vi "MultRRTPlan.vi"(7 "Parameters.lvclass":refnum<class "Parameters.lvclass">, 8 "Volta ao redor\nda área?":bool, 9 "Line?":bool, 10 "IA State":T7={"our_robots"=[], "enemy_robots"=[], "balls"=[], "geometry"={"line_width"=0, "field_length"=0, "field_width"=0, "boundary_width"=0, "referee_width"=0, "goal_width"=0, "goal_depth"=0, "goal_wall_width"=0, "center_circle_radius"=0, "defense_radius"=0, "defense_stretch"=0, "free_kick_from_defense_dist"=0, "penalty_spot_from_field_line_dist"=0, "penalty_line_from_spot_dist"=0}, "IA Judge"={"stage"="", "command"="", "our_goalie_id"=0.0, "enemy_goalie_id"=0.0, "command enum"=enum."Halt", "Time"=enum."Azul"}, "Received Timestamp"=timestamp(0 s since 1904-01-01), "Events"={"Touch"=FALSE, "Ball out"=FALSE, "id touch"=0.0, "Ball out of \nVision"=FALSE, "Ball inside \nGoalie area"=FALSE, "Robot not responding"=FALSE, "Robots responding status"=[1.0, 1.0, 1.0, 1.0, 1.0, 1.0], "Enemy Ball \nPossession"=FALSE, "Pass State"=FALSE, "id end of pass"=0.0, "Kick"=FALSE, "Id ini Possession"=0.0, "Ball Possesion"=FALSE, "Id Possesion"=0.0, "Direct Kick"=FALSE, "2nd Strk Ativo"=FALSE}}, 11 "Robot":T1={"id"=0, "function"=enum."Attacker", "x"=0.0, "y"=0.0, "orientation"=0.0, "v_tangent"=0.0, "v_normal"=0.0, "v_ang"=0.0, "kick_x"=0.0, "kick_z"=0.0, "dribble"=FALSE, "Timestamp"=timestamp(0 s since 1904-01-01), "estimatives"={"est_v_tangent"=0.0, "est_v_normal"=0.0, "est_vx"=0.0, "est_vy"=0.0, "Pos Robot Est"=[]}, "dest_x_kick"=0.0, "dest_y_kick"=0.0, "Gap Coord"=[], "States"=enum."GoToTangent", "Path "=[], "Path  Smooth"=[], "Dest"=[], "vx_desired"=0.0, "vy_desired"=0.0, "slowBehavior"=FALSE, "VSSStates"=enum."Pass"}) -> (2 "Robot Out":T1={"id"=0, "function"=enum."Attacker", "x"=0.0, "y"=0.0, "orientation"=0.0, "v_tangent"=0.0, "v_normal"=0.0, "v_ang"=0.0, "kick_x"=0.0, "kick_z"=0.0, "dribble"=FALSE, "Timestamp"=timestamp(0 s since 1904-01-01), "estimatives"={"est_v_tangent"=0.0, "est_v_normal"=0.0, "est_vx"=0.0, "est_vy"=0.0, "Pos Robot Est"=[]}, "dest_x_kick"=0.0, "dest_y_kick"=0.0, "Gap Coord"=[], "States"=enum."GoToTangent", "Path "=[], "Path  Smooth"=[], "Dest"=[], "vx_desired"=0.0, "vy_desired"=0.0, "slowBehavior"=FALSE, "VSSStates"=enum."Pass"})   [LabVIEW 2023]
uses:
  Vision_class/Old vision/Controls/AI Robot.ctl
  Vision_class/Old vision/Controls/Functions Enum.ctl
  Vision_class/Old vision/Controls/AttackerStates.ctl
  Vision_class/Old vision/Controls/PathDests.ctl
  Vision_class/Old vision/Controls/PathDest.ctl
  Navigation/VSSNavigation/VSSAttackerStates.ctl
  Vision_class/Old vision/SSL Detection Frame Simple Estimator Cameras VelCmd Folder/Core/AI Input.ctl
  Vision_class/Old vision/SSL Detection Frame Simple Estimator Cameras VelCmd Folder/Core/AI Ball.ctl
  Vision_class/Old vision/SSL Detection Frame Simple Estimator Cameras VelCmd Folder/Core/Field Size.ctl
  Vision_class/Old vision/SSL Detection Frame Simple Estimator Cameras VelCmd Folder/Core/AI Judge.ctl
  Communication_class/Paths/MessageAI_State Folder/Intel/Command Enum.ctl
  Vision_class/Old vision/SSL Detection Frame Simple Estimator Cameras VelCmd Folder/Util/Events/Events.ctl
  Parameters_class/Parameters.lvclass
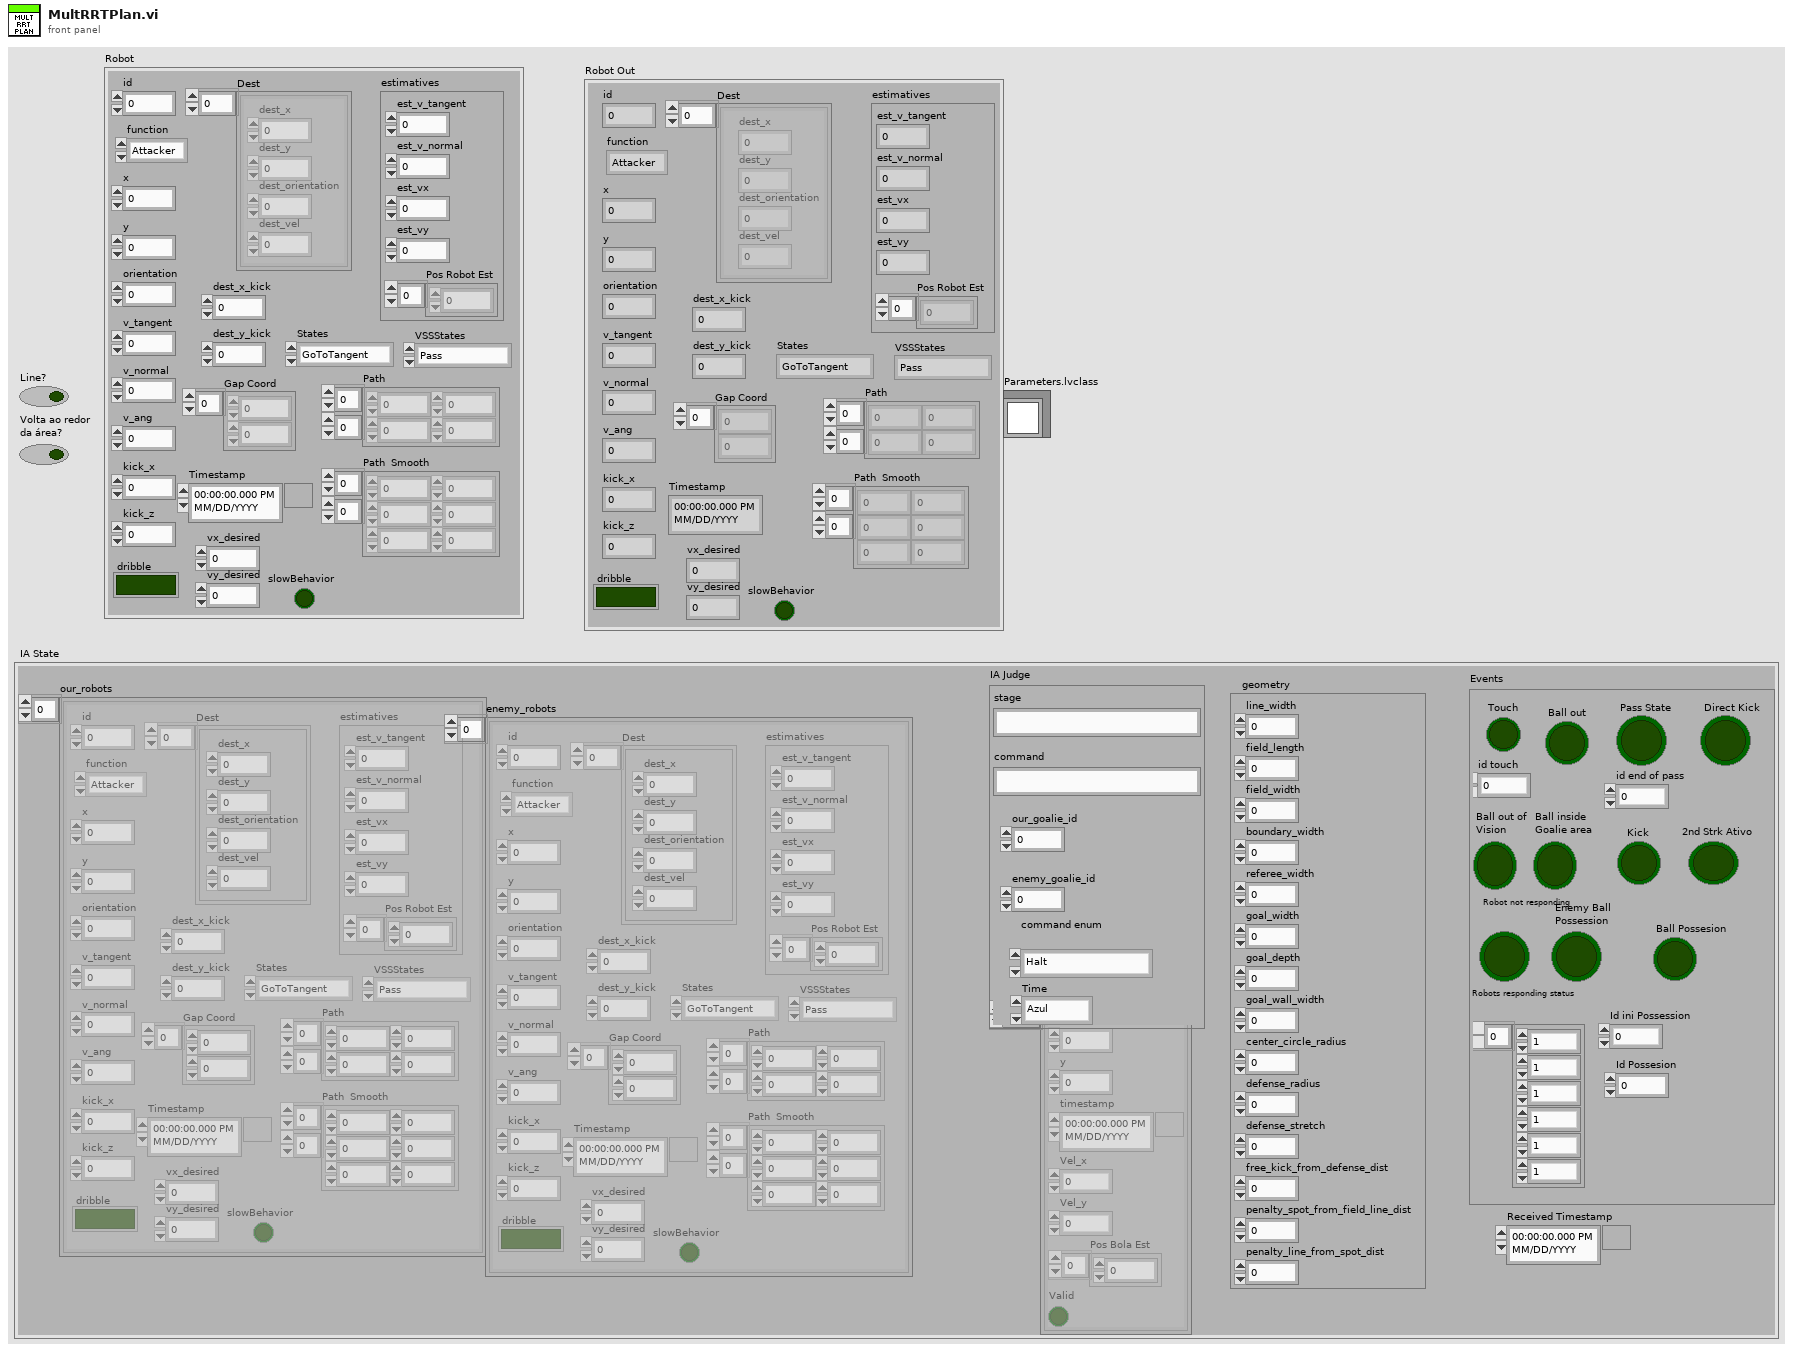
[diagram p1: front panel]
types:
  T1 = typedef "AI Robot.ctl" = cluster{"id":u32, "function":T2, "x":dbl, "y":dbl, "orientation":dbl, "v_tangent":dbl, "v_normal":dbl, "v_ang":dbl, "kick_x":dbl, "kick_z":dbl, "dribble":bool, "Timestamp":timestamp, "estimatives":cluster{"est_v_tangent":dbl, "est_v_normal":dbl, "est_vx":dbl, "est_vy":dbl, "Pos Robot Est":dbl[]}, "dest_x_kick":dbl, "dest_y_kick":dbl, "Gap Coord":dbl[], "States":T3, "Path ":dbl[][], "Path  Smooth":dbl[][], "Dest":T4, "vx_desired":dbl, "vy_desired":dbl, "slowBehavior":bool, "VSSStates":T6}
  T2 = typedef "Functions Enum.ctl" = enum16{"2nd Striker", "Attacker", "Goalie", "Defender", "Striker", "Goto 0", "Dummy", "Kicker", "ZigZag 0", "ZigZag 1", "ZigZag 2", "ZigZag 3", "ZigZag 4", "ZigZag 5", "ZigZag 6", "ZigZag 7", "ZigZag 8", ""}
  T3 = typedef "AttackerStates.ctl" = enum16{"Pass", "GoToTangent", "BallGetting", "GoToKick", ""}
  T4 = typedef "PathDests.ctl" = T5[]
  T5 = typedef "PathDest.ctl" = cluster{"dest_x":dbl, "dest_y":dbl, "dest_orientation":dbl, "dest_vel":dbl}
  T6 = typedef "VSSAttackerStates.ctl" = enum16{"Pass", "GoToTangent", "BallGetting", "GoToKick", "Rotate anti-clockwise", "Rotate Clockwise", ""}
  T7 = typedef "AI Input.ctl" = cluster{"our_robots":T1[], "enemy_robots":T1[], "balls":T8[], "geometry":T9, "IA Judge":T10, "Received Timestamp":timestamp, "Events":T12}
  T8 = typedef "AI Ball.ctl" = cluster{"x":dbl, "y":dbl, "timestamp":timestamp, "Vel_x":dbl, "Vel_y":dbl, "Pos Bola Est":dbl[], "Valid":bool}
  T9 = typedef "Field Size.ctl" = cluster{"line_width":u32, "field_length":u32, "field_width":u32, "boundary_width":u32, "referee_width":u32, "goal_width":u32, "goal_depth":u32, "goal_wall_width":u32, "center_circle_radius":u32, "defense_radius":u32, "defense_stretch":u32, "free_kick_from_defense_dist":u32, "penalty_spot_from_field_line_dist":u32, "penalty_line_from_spot_dist":u32}
  T10 = typedef "AI Judge.ctl" = cluster{"stage":string, "command":string, "our_goalie_id":dbl, "enemy_goalie_id":dbl, "command enum":T11, "Time":enum16{"Azul", "Amarelo"}}
  T11 = typedef "Command Enum.ctl" = enum16{"Halt", "Stop", "Force Start", "PKA Normal Start", "Prepare Kickoff Ally", "PKE Normal Start", "Prepare Kickoff Enemy", "Prepare Penalty Ally", "PPA Normal Start", "Prepare Penalty Enemy", "PPE Normal Start", "Direct Free Enemy", "Direct Free Ally", "Indirect Free Enemy", "Indirect Free Ally", "Timeout Enemy", "Timeout Ally", "Goal Enemy", "Goal Ally", "Ball Placement Enemy", "Ball Placement Ally", "Normal Half Time", "Extra Time Break", "Extra Half Time", "None", "Post Game"}
  T12 = typedef "Events.ctl" = cluster{"Touch":bool, "Ball out":bool, "id touch":dbl, "Ball out of \nVision":bool, "Ball inside \nGoalie area":bool, "Robot not responding":bool, "Robots responding status":dbl[], "Enemy Ball \nPossession":bool, "Pass State":bool, "id end of pass":dbl, "Kick":bool, "Id ini Possession":dbl, "Ball Possesion":bool, "Id Possesion":dbl, "Direct Kick":bool, "2nd Strk Ativo":bool}
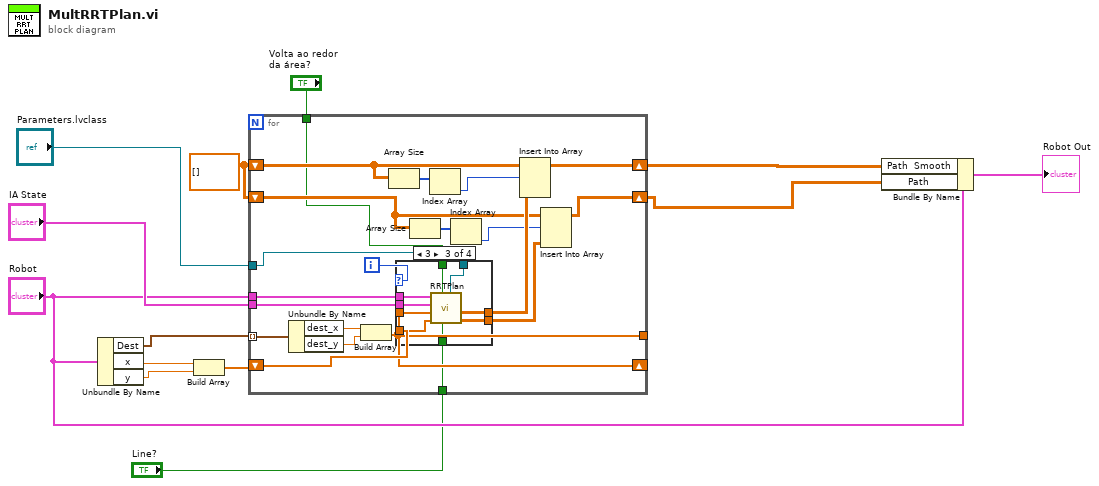
[diagram p0: block diagram]
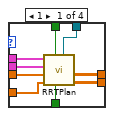
[diagram p2: hidden frame]
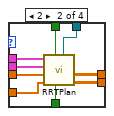
[diagram p3: hidden frame]
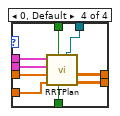
[diagram p4: hidden frame]
diagram:
  w8 = dbl[][] [] ("Path")
  n1 = Unbundle By Name("Robot") -> ("Dest"=w6:T4, "x"=w13:dbl, "y"=w12:dbl)
  n2 = Build Array(w13, w12) -> (w9:dbl[])
  n3 = for {
    tunnel: "Robot" -> [w33]
    tunnel: "IA State" -> [w34]
    shift-right: [w27] -> w4
    shift-left: w8 -> [w26]
    tunnel: w6 -> [w32] mode=indexing
    shift-right: [w23] -> _
    shift-left: w9 -> [w29]
    tunnel: [w23] -> _
    shift-right: [w19] -> w5
    shift-left: w8 -> [w20]
    tunnel: "Line?" -> [w16]
    tunnel: "Volta ao redor\nda área?" -> [w15]
    tunnel: "Parameters.lvclass" -> [w14]
    i -> [w17]
    n4 = Unbundle By Name(w32) -> ("dest_x"=w31:dbl, "dest_y"=w30:dbl)
    n5 = Build Array(w31, w30) -> (w23:dbl[])
    n6 = Array Size(array=w26) -> (size(s)=w25:i32[])
    n7 = case shown="3" w17 {
      tunnel: w34 -> [w43 w52 w61 w70]
      tunnel: w33 -> [w42 w51 w60 w69]
      tunnel: w29 -> [w41 w50 w59 w68]
      tunnel: [w40 w49 w58 w67] -> w28
      tunnel: w23 -> [w39 w48 w57 w66]
      tunnel: [w38 w47 w56 w65] -> w18
      tunnel: w16 -> [w37 w46 w55 w64]
      tunnel: w15 -> [w36 w45 w54 w63]
      tunnel: w14 -> [w35 w44 w53 w62]
      frame 1 {
        n8 = call "RRTPlan.vi"("Parameters.lvclass"=w35, "Line?"=w37, "Volta ao redor\nda área?"=w36, "Initial Pos x,y"=w41, "Dest x,y"=w39, "IA State"=w43, "Robot"=w42) -> ("Path"=w38:dbl[][], "Smooth Path"=w40:dbl[][])  [unwired: 3 in]
      }
      frame 2 {
        n9 = call "RRTPlan.vi"("Parameters.lvclass"=w44, "Line?"=w46, "Volta ao redor\nda área?"=w45, "Initial Pos x,y"=w50, "Dest x,y"=w48, "IA State"=w52, "Robot"=w51) -> ("Path"=w47:dbl[][], "Smooth Path"=w49:dbl[][])  [unwired: 3 in]
      }
      frame 3 {
        n10 = call "RRTPlan.vi"("Parameters.lvclass"=w53, "Line?"=w55, "Volta ao redor\nda área?"=w54, "Initial Pos x,y"=w59, "Dest x,y"=w57, "IA State"=w61, "Robot"=w60) -> ("Path"=w56:dbl[][], "Smooth Path"=w58:dbl[][])  [unwired: 3 in]
      }
      frame 0, Default {
        n11 = call "RRTPlan.vi"("Parameters.lvclass"=w62, "Line?"=w64, "Volta ao redor\nda área?"=w63, "Initial Pos x,y"=w68, "Dest x,y"=w66, "IA State"=w70, "Robot"=w69) -> ("Path"=w65:dbl[][], "Smooth Path"=w67:dbl[][])  [unwired: 3 in]
      }
    }
    n12 = Array Size(array=w20) -> (size(s)=w21:i32[])
    n13 = Index Array(array=w25) -> (element=w24:i32)  [unwired: 1 in]
    n14 = Index Array(array=w21) -> (element=w22:i32)  [unwired: 1 in]
    n15 = Insert Into Array(array=w26, index (row)=w24, new element=w28) -> (w27:dbl[][])  [unwired: 1 in]
    n16 = Insert Into Array(array=w20, index (row)=w22, new element=w18) -> (w19:dbl[][])  [unwired: 1 in]
  }
  n17 = Bundle By Name(cluster="Robot", "Path  Smooth"=w4, "Path"=w5) -> (→"Robot Out":T1)
